vi "Get gRPC Id Terminal For Event SubDiagram.vi"(10 "Frame Index in":i32, 11 "Event Structure ref in":refnum<vi>) -> (3 "Term Refnum":refnum<vi>)   [LabVIEW 2019, in "gRPC Template Creation Utility.lvlib"]
uses:
  gRPC Template Creation Utility.lvlib
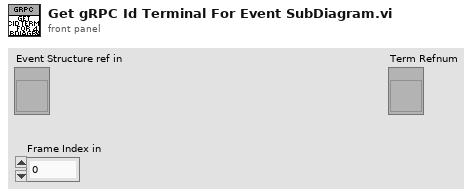
[diagram p1: front panel]
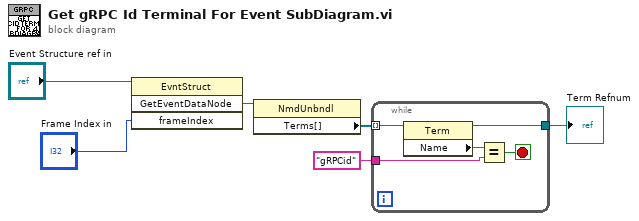
[diagram p0: block diagram]
diagram:
  n1 = invoke class="EvntStruct" method="GetEventDataNode"(reference="Event Structure ref in", "frameIndex"="Frame Index in") -> ("GetEventDataNode"=w6:refnum<vi>)  [unwired: 2 in, 3 out]
  n2 = property class="NmdUnbndl"(reference=w6) -> ("Terms[]"=w5:refnum<vi>[])  [unwired: 1 in, 2 out]
  n3 = while {
    tunnel: w5 -> [w11] mode=indexing
    tunnel: [w10] -> w1
    tunnel: "gRPCid" -> [w8]
    stop <- w7 stop-if-true
    n4 = property class="Term"(reference=w11) -> (reference out=w10:refnum<vi>, "Name"=w9:string)  [unwired: 1 in, 1 out]
    n5 = Equal?(x=w9, y=w8) -> (x = y?=w7:bool)
  }
  "Term Refnum" <- w1
